vi "SubVI_Read_Write_EEG.vi"(8 "error in (no error)":errorcluster, 10 "LINX Resource in":T1, 11 "Weight Array":i32[](array[numeric])) -> (0 "error out":errorcluster, 2 "LINX Resource out 2":T1, 3 "Raw EEG out":T7)   [LabVIEW 2020]
uses:
  <vilib>/MakerHub/LINX/Private/Type Defs/LINX Ref.ctl
  <vilib>/MakerHub/LINX/Private/Type Defs/Platform.ctl
  <vilib>/MakerHub/LINX/Private/Type Defs/Interface.ctl
  <vilib>/MakerHub/LINX/Private/Device/Type Defs/LINX Device Config.ctl
  <vilib>/MakerHub/LINX/Private/Device/Type Defs/TCP Config.ctl
  <vilib>/MakerHub/LINX/Private/Device/Type Defs/Channels.ctl
  <extravilib>/ChannelInstances/Lossy Stream-a[.](dbl)/)Channel.ctl
  <vilib>/MakerHub/LINX/Private/Type Defs/Peripherals/SPI/SPI Configuration.ctl
  <vilib>/MakerHub/LINX/Private/Type Defs/Peripherals/SPI/SPI Bit Order.ctl
  <vilib>/MakerHub/LINX/Private/Type Defs/Peripherals/SPI/SPI Mode.ctl
  <vilib>/MakerHub/LINX/Public/Peripherals/SPI/SPI CS Config.ctl
  <vilib>/MakerHub/LINX/Private/Type Defs/Peripherals/SPI/SPI CS Logic Level.ctl
  <vilib>/MakerHub/LINX/Public/Peripherals/SPI/SPI Write Read 1 Frame.vi
  <vilib>/MakerHub/LINX/Public/Peripherals/SPI/SPI Write Read N Frames.vi
  <extravilib>/ChannelInstances/Lossy Stream-a[.](dbl)/Endpoint.vi
  <vilib>/MakerHub/LINX/Private/Local IO/LinxSpiWriteRead.vi
  <vilib>/MakerHub/LINX/Public/Utilities/Check Channel.vi
  <vilib>/MakerHub/LINX/Private/Local IO/Handle Errors.vi
  Global 1.vi
  <vilib>/MakerHub/LINX/Private/Utilties/Generate Error.vi
  <extravilib>/ChannelInstances/Lossy Stream-a[.](dbl)/)Channel.vi
  <vilib>/MakerHub/LINX/LMH-LINX.lvlib
  <extravilib>/ChannelInstances/Lossy Stream-a[.](dbl).lvlib
  <vilib>/MakerHub/LINX/Private/Device/Device.lvlib
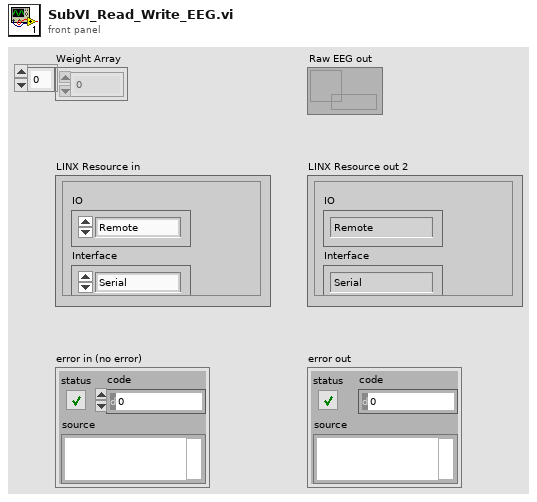
[diagram p1: front panel]
types:
  T1 = typedef "LMH-LINX.lvlib/LINX Ref.ctl" = cluster{"IO":T2, "Interface":T3, "LINX Device Config":T4}
  T2 = typedef "LMH-LINX.lvlib/Platform.ctl" = enum16{"Remote", "Local"}
  T3 = typedef "LMH-LINX.lvlib/Interface.ctl" = enum16{"Serial", "TCP"}
  T4 = typedef "LMH-LINX.lvlib/Device.lvlib/LINX Device Config.ctl" = cluster{"Interface":T3, "COM Port":refnum<visa-resource-name>, "TCP Configuration":T5, "Device Family":u8, "Device ID":u8, "Device Name":string, "TCP Ref":refnum<k5>, "Channels":T6}
  T5 = typedef "LMH-LINX.lvlib/Device.lvlib/TCP Config.ctl" = cluster{"IP Address":string, "Port":u16}
  T6 = typedef "LMH-LINX.lvlib/Channels.ctl" = cluster{"DI":u8[], "DO":u8[], "AI":u8[], "AO":u8[], "PWM":u8[], "QE":u8[], "UART":u8[], "I2C 2":u8[], "SPI":u8[], "CAN":u8[], "Servo":u8[], "AI Ref (V)":dbl, "AI Resolution (Bits)":u8, "AO Ref (V)":dbl, "AO Resolution (Bits)":u8}
  T7 = typedef "Lossy Stream-a[.](dbl).lvlib/)Channel.ctl" = refnum<queue>
  T8 = typedef "LMH-LINX.lvlib/SPI CS Config.ctl" = cluster{"CS Channel":u8, "CS Logic Level":T9}
  T9 = typedef "LMH-LINX.lvlib/SPI CS Logic Level.ctl" = enum8{"Active Low", "Active High"}
  T10 = typedef "LMH-LINX.lvlib/SPI Configuration.ctl" = cluster{"Clock Frequency":u32, "Bit Order":T11, "SPI Mode":T12}
  T11 = typedef "LMH-LINX.lvlib/SPI Bit Order.ctl" = enum8{"LSb First", "MSb First"}
  T12 = typedef "LMH-LINX.lvlib/SPI Mode.ctl" = enum8{"Mode 0", "Mode 1", "Mode 2", "Mode 3"}
  T13 = typedef "LVDateTimeRec.ctl" = cluster{"fractional second":dbl, "second":i32, "minute":i32, "hour":i32, "day of month":i32, "month":i32, "year":i32, "day of week":i32, "day of year":i32, "DST":i32}
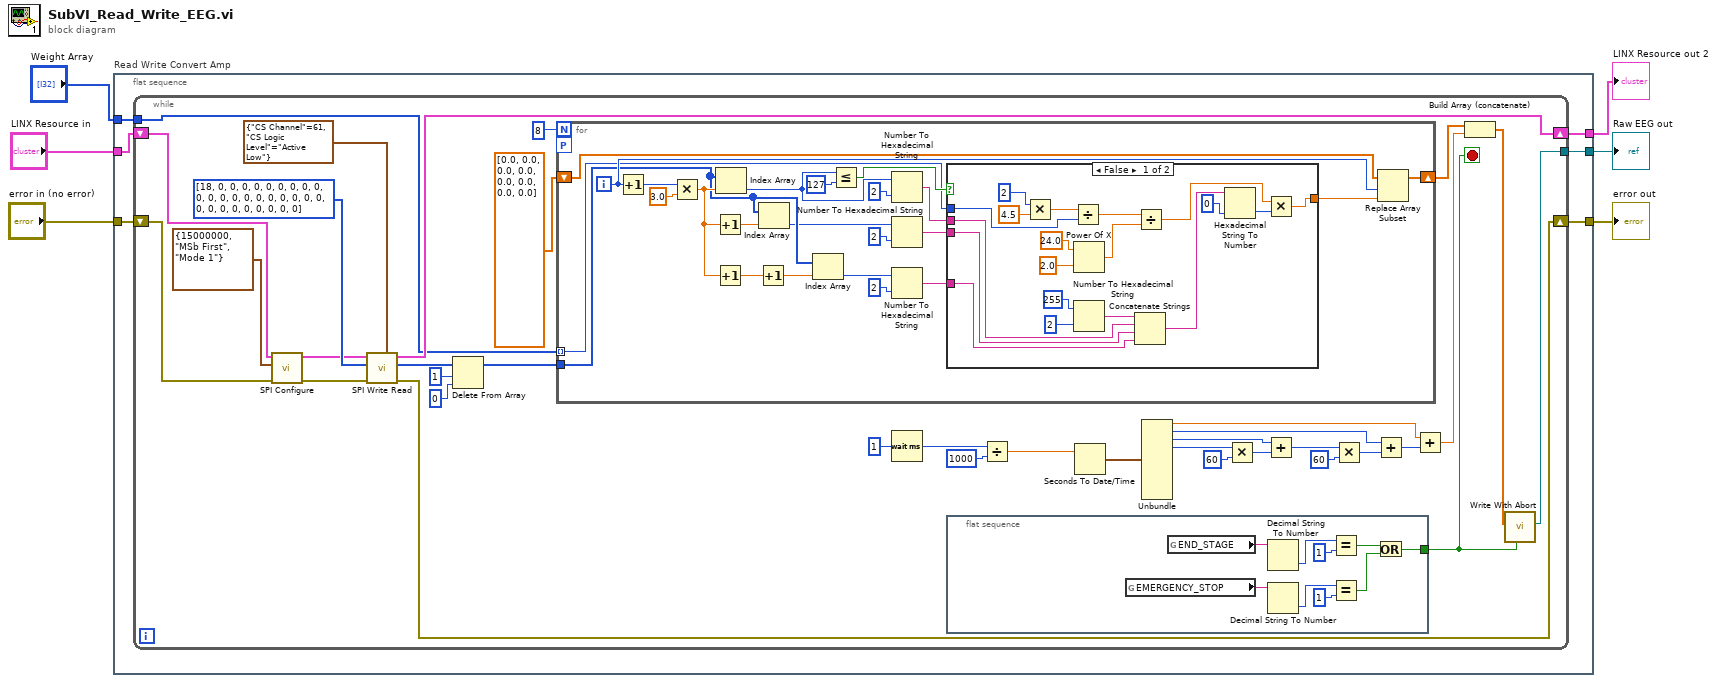
[diagram p0: block diagram]
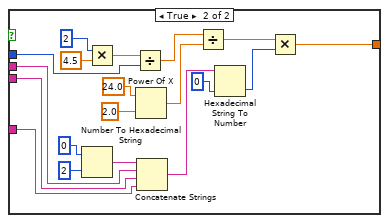
[diagram p2: hidden frame]
diagram:
  n1 = flat-sequence "Read Write Convert Amp" {
    tunnel: [w12] -> w1
    tunnel: [w11] -> w2
    tunnel: [w10] -> w3
    tunnel: "error in (no error)" -> [w9]
    tunnel: "LINX Resource in" -> [w8]
    tunnel: "Weight Array" -> [w7]
    frame #0 {
      n2 = while {
        shift-right: [w47] -> w11
        shift-left: w9 -> [w46]
        shift-right: [w45] -> w12
        shift-left: w8 -> [w48]
        tunnel: [w44] -> w10
        tunnel: w7 -> [w43]
        stop <- w42 stop-if-true
        n3 = call <vilib>:"SPI Configure.vi"("Error In"=w46, "SPI Configuration"=T10 {"Clock Frequency"=15000000, "Bit Order"=enum."MSb First", "SPI Mode"=enum."Mode 1"}, "LINX Resource"=w48) -> ("Error Out"=w38:errorcluster, "LINX Resource"=w37:T1)  [unwired: 6 in, 1 out]
        n4 = call-poly <vilib>:"SPI Write Read.vi"("CS Configuration"=T8 {"CS Channel"=61, "CS Logic Level"=enum."Active Low"}, "Error In"=w38, "Data"=u8[] [18, 0, 0, 0, 0, 0, 0, 0, 0, 0, 0, 0, 0, 0, 0, 0, 0, 0, 0, 0, 0, 0, 0, 0, 0, 0, 0, 0, 0, 0], "LINX Resource"=w37) -> ("Error Out"=w47:errorcluster, "Read Data"=w18:u8[], "LINX Resource"=w45:T1)  [unwired: 4 in, 1 out]
        n5 = Delete From Array(array=w18, length=1, index=0) -> (array with subset deleted=w17:u8[])  [unwired: 1 out]
        n6 = for {
          N: 8 -> [_]
          shift-right: [w54] -> w14
          shift-left: dbl[] [0.0, 0.0, 0.0, 0.0, 0.0, 0.0, 0.0, 0.0] -> [w55]
          tunnel: w17 -> [w52]
          tunnel: w43 -> [w53] mode=indexing
          workers-P: _ -> [_]
          i -> [w56]
          n7 = Increment(x=w56) -> (x+1=w62:i32)
          n8 = Multiply(x=w62, y=3.0) -> (x*y=w61:dbl)
          n9 = Increment(x=w61) -> (x+1=w58:dbl)
          n10 = Increment(x=w61) -> (x+1=w59:dbl)
          n11 = Index Array(array=w52, index=w61) -> (element=w49:u8)
          n12 = Increment(x=w59) -> (x+1=w60:dbl)
          n13 = Index Array(array=w52, index=w58) -> (element=w50:u8)
          n14 = Index Array(array=w52, index=w60) -> (element=w51:u8)
          n15 = Less Or Equal?(x=w49, y=u8 127) -> (x <= y?=w70:bool)
          n16 = Number To Hexadecimal String(1:i16 2 ("width (-)"), 2:w49) -> (0:w67:string)
          n17 = Number To Hexadecimal String(1:i16 2 ("width (-)"), 2:w50) -> (0:w68:string)
          n18 = Number To Hexadecimal String(1:i16 2 ("width (-)"), 2:w51) -> (0:w69:string)
          n19 = case shown="False" w70 {
            tunnel: w69 -> [w81 w99]
            tunnel: w68 -> [w82 w98]
            tunnel: w67 -> [w83 w97]
            tunnel: [w77 w96] -> w57
            tunnel: w53 -> [w72 w91]
            frame False {
              n20 = Multiply(x=2, y=4.5) -> (x*y=w88:dbl)
              n21 = Divide(x=w88, y=w72) -> (x/y=w85:dbl)
              n22 = Power Of X(1:2.0 ("x"), 2:24.0 ("y")) -> (0:w84:dbl)
              n23 = Number To Hexadecimal String(1:i16 2 ("width (-)"), 2:255) -> (0:w79:string)
              n24 = Concatenate Strings(w79, w83, w82, w81) -> (w75:string)
              n25 = Divide(x=w85, y=w84) -> (x/y=w78:dbl)
              n26 = Hexadecimal String To Number(string=w75, default (0uL)=0 ("default (0 U32)")) -> (number=w74:i32)  [unwired: 1 in, 1 out]
              n27 = Multiply(x=w78, y=w74) -> (x*y=w77:dbl)
            }
            frame True {
              n28 = Number To Hexadecimal String(1:i16 2 ("width (-)"), 2:0) -> (0:w101:string)
              n29 = Multiply(x=2, y=4.5) -> (x*y=w107:dbl)
              n30 = Divide(x=w107, y=w91) -> (x/y=w104:dbl)
              n31 = Power Of X(1:2.0 ("x"), 2:24.0 ("y")) -> (0:w103:dbl)
              n32 = Concatenate Strings(w101, w97, w98, w99) -> (w94:string)
              n33 = Divide(x=w104, y=w103) -> (x/y=w100:dbl)
              n34 = Hexadecimal String To Number(string=w94, default (0uL)=0 ("default (0 U32)")) -> (number=w95:i32)  [unwired: 1 in, 1 out]
              n35 = Multiply(x=w100, y=w95) -> (x*y=w96:dbl)
            }
          }
          n36 = Replace Array Subset(array=w55, new element=w57, index=w56) -> (w54:dbl[])
        }
        n37 = Wait (ms)(milliseconds to wait=u32 1) -> (millisecond timer value=w33:u32)
        n38 = flat-sequence {
          tunnel: [w110] -> w42
          frame #0 {
            n39 = global read "Global 1.vi" "EMERGENCY_STOP"() -> (w113:string)
            n40 = global read "Global 1.vi" "END_STAGE"() -> (w118:string)
            n41 = Decimal String To Number(string=w118) -> (number=w117:i32)  [unwired: 2 in, 1 out]
            n42 = Decimal String To Number(string=w113) -> (number=w115:i32)  [unwired: 2 in, 1 out]
            n43 = Equal?(x=w117, y=1) -> (x = y?=w111:bool)
            n44 = Equal?(x=w115, y=1) -> (x = y?=w112:bool)
            n45 = Or(x=w111, y=w112) -> (x .or. y?=w110:bool)
          }
        }
        n46 = Divide(x=w33, y=u32 1000) -> (x/y=w34:dbl)
        n47 = Seconds To Date/Time(time stamp (now)=w34) -> (date time rec=w32:T13)  [unwired: 1 in]
        n48 = Unbundle(w32) -> ("fractional second"=w22:dbl, "second"=w23:i32, "minute"=w25:i32, "hour"=w27:i32)  [unwired: 6 out]
        n49 = Multiply(x=w27, y=60) -> (x*y=w31:i32)
        n50 = Add(x=w25, y=w31) -> (x+y=w30:i32)
        n51 = Multiply(x=w30, y=60) -> (x*y=w29:i32)
        n52 = Add(x=w23, y=w29) -> (x+y=w28:i32)
        n53 = Add(x=w22, y=w28) -> (x+y=w13:dbl)
        n54 = Build Array (concatenate)(w14, w13) -> (w21:dbl[])
        n55 = call <extravilib>:"Write With Abort.vi"("abort"=w42, "element"=w21) -> ("channel"=w44:T7)  [unwired: 6 in, 3 out]
      }
    }
  }
  "Raw EEG out" <- w3
  "error out" <- w2
  "LINX Resource out 2" <- w1
